vi "SendCfgFileWebDAV.vi"(3 "error in":errorcluster caption="entrée d'erreur (pas d'erreur)", 5 "NomProjet":string) -> (0 "error out":errorcluster caption="sortie d'erreur", 2 "NomProjetOut":string)   [LabVIEW 2015]
uses:
  DefDeType/WhichPath.ctl
  <vilib>/WebDAVClient/Simple Put File.vi
  <vilib>/WebDAVClient/NI_WebDAV.lvlib
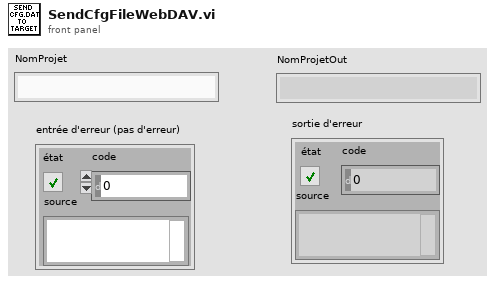
[diagram p1: front panel]
types:
  T1 = typedef "WhichPath.ctl" = enum16{"DossierProjet", "Config", "Meas", "MeasSuitCase", "MeasOnBoard", "MeasQualisys", "MeasTDMS", "MeasHexapode", "Fig", "Res"}
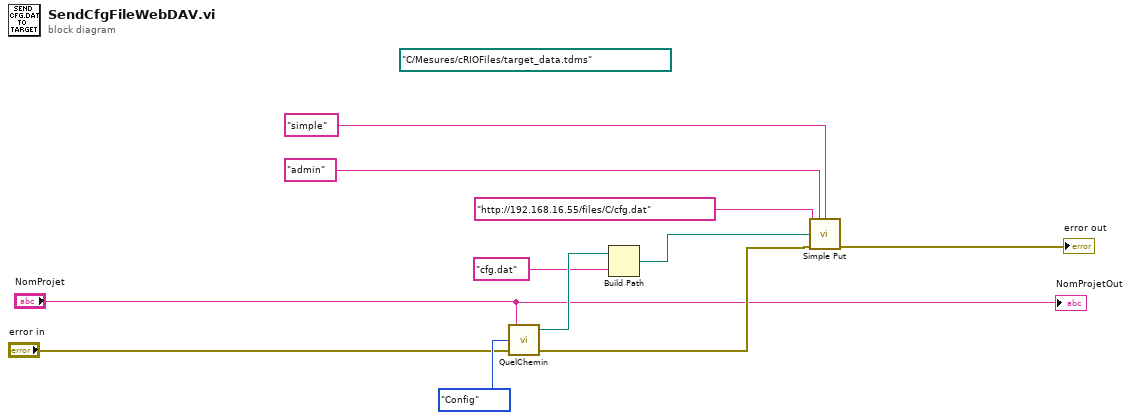
[diagram p0: block diagram]
diagram:
  (unwired) path "C:/Mesures/cRIOFiles/target_data.tdms" ("local file path")
  n1 = call "QuelChemin.vi"("Entrée d'erreur"="error in", "WhichPath?"=WhichPath."Config", "NomProjet"="NomProjet") -> ("Sortie d'erreur"=w7:errorcluster, "SurDisqueLocal"=w5:path)  [unwired: 1 out]
  n2 = Build Path(base path=w5, name or relative path="cfg.dat" ("username")) -> (appended path=w3:path)
  n3 = call-poly <vilib>:"Simple Put.vi"("file uri"="http://192.168.16.55/files/C/cfg.dat" ("remote file uri"), "username"="admin", "password"="simple", "local file path"=w3, "error in (no error)"=w7) -> ("error out"=→"error out":errorcluster)  [unwired: 9 in, 1 out]
  "NomProjetOut" <- "NomProjet"
